vi "NISE.remote.Write ActiveNVMEMArea.vi"(8 "error in (no error)":errorcluster, 10 "ActiveNVMEMArea":refnum<k21>, 11 "SLSC Remote in":refnum<class "SLSC Interface.lvclass">) -> (0 "error out":errorcluster, 3 "SLSC Remote out":refnum<class "SLSC Interface.lvclass">)   [LabVIEW 2016, in "SLSC Interface.lvclass"]
uses:
  SLSC Interface Class/SLSC Interface.lvclass
  <vilib>/NI/JSON Support for LabVIEW/JSON Data Classes/JSON String/JSON String.lvclass
  C:/Program Files (x86)/National Instruments/LabVIEW 2016/vi.lib/NI/JSON Support for LabVIEW/JSON Data Classes/JSON Datatype/JSON Null.lvclass
  <vilib>/NI/JSON Support for LabVIEW/JSON Data Classes/JSON String/New JSON String.vi
  <vilib>/NI/JSON Support for LabVIEW/JSON Data Classes/JSON Helper/JSON Helper.lvclass
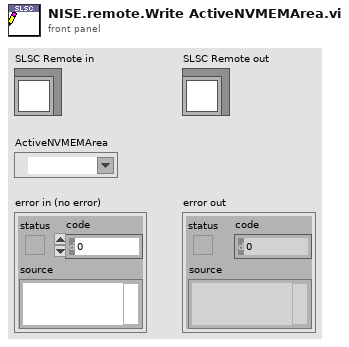
[diagram p1: front panel]
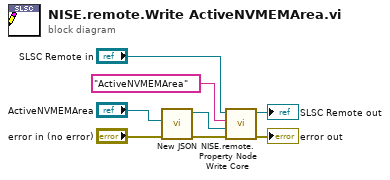
[diagram p0: block diagram]
diagram:
  n1 = call-poly <vilib>:"New JSON.vi"("error in (no error)"="error in (no error)", "value"="ActiveNVMEMArea") -> ("error out"=w2:errorcluster, "JSON String out"=w1:refnum<class "JSON String.lvclass">)  [unwired: 8 in]
  n2 = call "NISE.remote.Property Node Write Core.vi"("error in (no error)"=w2, "value"=w1, "property"="ActiveNVMEMArea", "SLSC Remote in"="SLSC Remote in") -> ("error out"=→"error out":errorcluster, "SLSC Remote out"=→"SLSC Remote out":refnum<class "SLSC Interface.lvclass">)  [unwired: 6 in]
